vi "Remove Constant Current 3.vi"(3 "error in":errorcluster) -> (10 "error out":errorcluster)   [LabVIEW 2015]
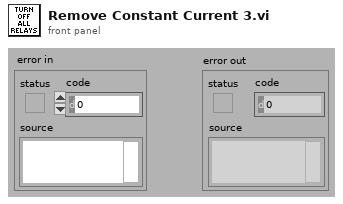
[diagram p1: front panel]
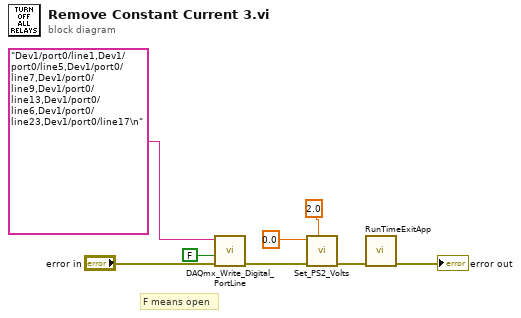
[diagram p0: block diagram]
diagram:
  # "F means open"
  n1 = call "DAQmx_Write_Digital_PortLine.vi"("Device/Ports/Lines"="Dev1/port0/line1,Dev1/port0/line5,Dev1/port0/line7,Dev1/port0/line9,Dev1/port0/line13,Dev1/port0/line6,Dev1/port0/line23,Dev1/port0/line17\n", "Boolean"=FALSE, "error in"="error in") -> ("error out"=w4:errorcluster)  [unwired: 6 in, 1 out]
  n2 = call "Set_PS2_Volts.vi"("Output Voltage"=0.0 ("Output Voltage (0)"), "error in"=w4, "delay (secs)"=2.0 ("Output Voltage (0)")) -> ("error out"=w3:errorcluster)  [unwired: 5 in, 2 out]
  n3 = call "RunTimeExitApp.vi"("error in (no error)"=w3) -> ("error out"=→"error out":errorcluster)  [unwired: 10 in]
